vi "Map Generator.vi"(1 "NxN":i32) -> (0 "Map":i32[][](array[numeric]))   [LabVIEW 2015]
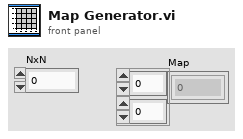
[diagram p1: front panel]
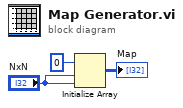
[diagram p0: block diagram]
diagram:
  n1 = Initialize Array(0 ("dimension size"), "NxN", "NxN") -> (→"Map":i32[][])
